vi "init.vi"(8 "error in (no error)":errorcluster, 11 "NotifierStopMechanism in":refnum<class "BoolNotifierStopMechanism.lvclass">) -> (0 "error out":errorcluster, 3 "NotifierStopMechanism out":refnum<class "BoolNotifierStopMechanism.lvclass">)   [LabVIEW 2023, in "TLC_Daemon.lvlib" / "BoolNotifierStopMechanism.lvclass"]
doc: "Initializes the stop mechanism.\n_____________________________________\nTLC Daemon 1.0.0.2\nCopyright (c) 2026 Andrea Cadei"
uses:
  BoolNotifierStopMech/BoolNotifierStopMechanism.lvclass
  BoolNotifierStopMech/BoolNotifierStopMechanism.lvclass/BoolNotifierStopMechanism.ctl
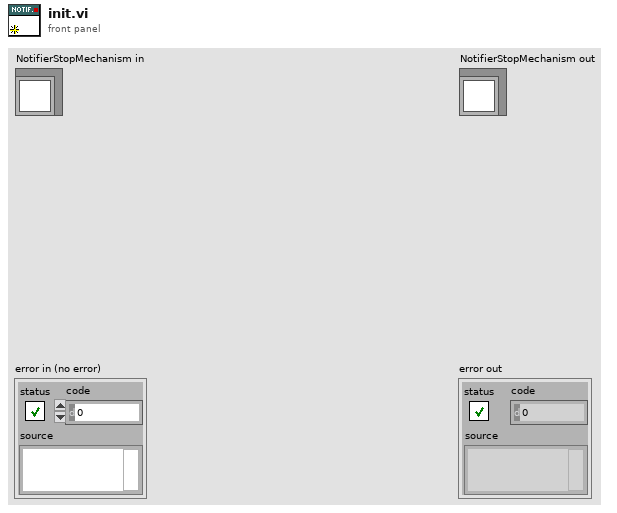
[diagram p1: front panel]
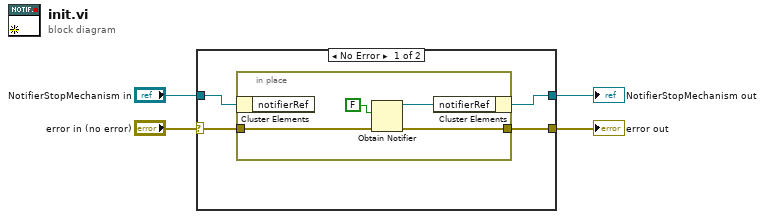
[diagram p0: block diagram]
diagram:
  n1 = case shown="No Error" "error in (no error)" {
    selector: "error in (no error)" -> [w8 w14]
    tunnel: [w7 w14] -> w4
    tunnel: [w5 w13] -> w1
    tunnel: "NotifierStopMechanism in" -> [w6 w13]
    frame No Error {
      n2 = in-place {
        in-place-border: w8 -> [w11]
        in-place-border: [w10] -> w7
        n3 = in-place-cluster #1(w6) -> ()  [unwired: 1 out]
        n4 = Obtain Notifier(notification data type=FALSE, error in (no error)=w11) -> (notifier out=w9:refnum<notifier>, error out=w10:errorcluster)  [unwired: 2 in, 1 out]
        n5 = in-place-cluster #1("notifierRef"=w9) -> (w5:refnum<class "BoolNotifierStopMechanism.lvclass">)
      }
    }
    frame Error {
    }
  }
  "error out" <- w4
  "NotifierStopMechanism out" <- w1
